vi "get status .vi"(11 "para0":u32) -> (2 "function return":i32, 3 "para0 out":u32)   [LabVIEW 2020, in "cDaq.lvlib"]
doc: "DAQAPI int get_status_(HDAQ);"
uses:
  cDaq.lvlib
  cDaq.dll
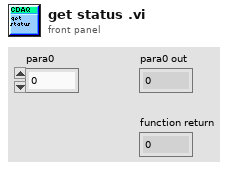
[diagram p1: front panel]
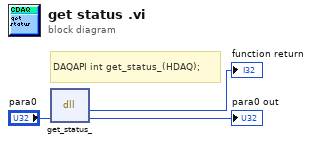
[diagram p0: block diagram]
diagram:
  # "DAQAPI int get_status_(HDAQ);"
  n1 = dll-call lib="G:/CODE/01-Cplusplus/cDaq/doc/UsingWithLabview/cDaqlib/cDaq.*" fn="get_status_"("para0"="para0") -> (→"function return":i32, "para0"=→"para0 out":u32)  [unwired: 3 in, 2 out]
